vi "Test_Pass.vi"(11 "Test Case In":refnum<class "Broken Test.lvclass">) -> (0 "error out":errorcluster, 3 "Test Case Out":refnum<class "Broken Test.lvclass">)   [LabVIEW 2020, in "Broken Test.lvclass"]
uses:
  Broken Test.lvclass
  Broken Test.lvclass/Broken Test.ctl
  4acd223d-b712-4434-8bc5-6d2ce5207c44.vi
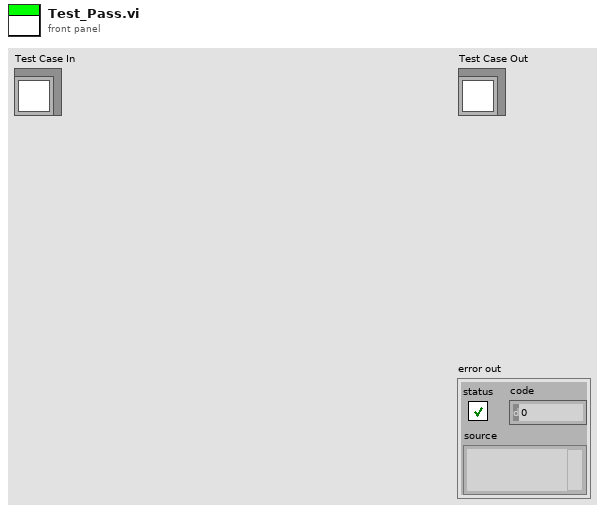
[diagram p1: front panel]
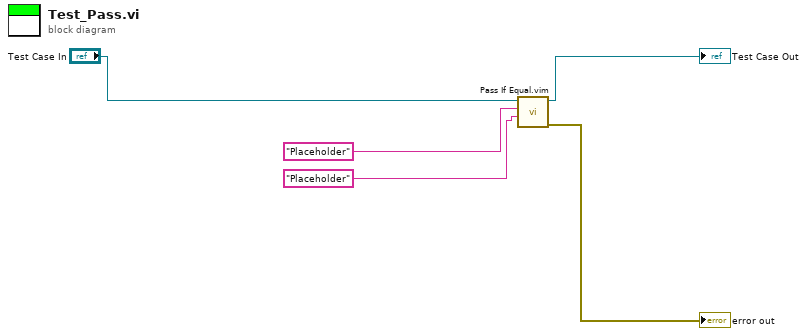
[diagram p0: block diagram]
diagram:
  n1 = call "Pass If Equal.vim"("Actual"="Placeholder", "Expected"="Placeholder", "LUnit Test Case In"="Test Case In") -> ("error out"=→"error out":errorcluster, "LUnit Test Case Out"=→"Test Case Out":refnum<class "Broken Test.lvclass">)  [unwired: 7 in]
